vi "CloseTrig.vi"(8 "error in (no error)":errorcluster, 10 "ClkName":string, 11 "NiPxi6682 in":refnum<class "NiPxi6682.lvclass">) -> (0 "error out":errorcluster, 3 "NiPxi6682 out":refnum<class "NiPxi6682.lvclass">)   [LabVIEW 2014, in "SyncPlugins.lvlib" / "NiPxi6682.lvclass"]
uses:
  NiPxi6682.lvclass
  SyncPluginBase/SyncPluginBase.lvclass
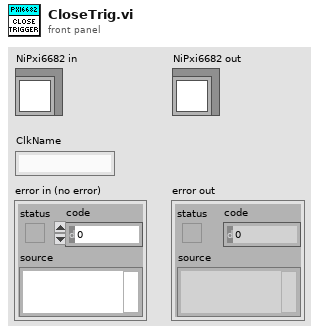
[diagram p1: front panel]
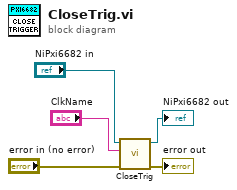
[diagram p0: block diagram]
diagram:
  n1 = call-parent "CloseTrig.vi"("error in (no error)"="error in (no error)", "ClkName"="ClkName", "SyncPluginBase in"="NiPxi6682 in") -> ("error out"=→"error out":errorcluster, "SyncPluginBase out"=→"NiPxi6682 out":refnum<class "NiPxi6682.lvclass">)  [unwired: 7 in]
